vi "ExtractVINames.vi"(8 "error in (no error)":errorcluster, 11 "vi paths":string[](array[string])) -> (0 "error out":errorcluster, 3 "vi names":string[](array[string]))   [LabVIEW 2015, in "VeriStandTestUtilities.lvlib"]
uses:
  VeriStandTestUtilities.lvlib
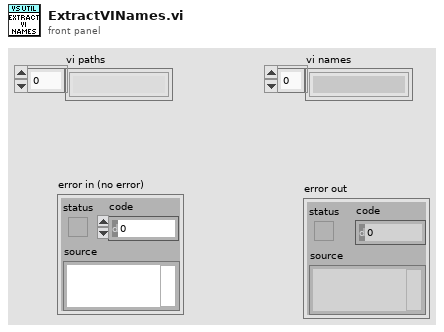
[diagram p1: front panel]
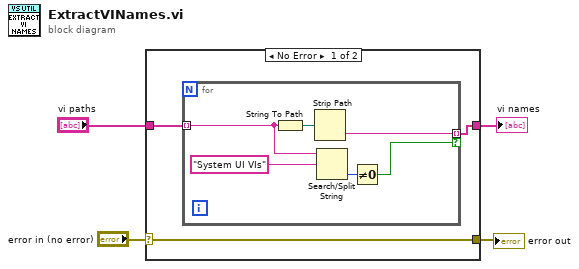
[diagram p0: block diagram]
diagram:
  n1 = case shown="No Error" "error in (no error)" {
    selector: "error in (no error)" -> [w5 w15]
    tunnel: [w5 w15] -> w4
    tunnel: "vi paths" -> [w7 w14]
    tunnel: [w6 w14] -> w1
    frame No Error {
      n2 = for {
        tunnel: w7 -> [w10] mode=indexing
        tunnel: [w9] -> w6 mode=indexing if=w8
        n3 = String To Path(string=w10) -> (path=w13:path)
        n4 = Strip Path(path=w13) -> (name=w9:string)  [unwired: 1 out]
        n5 = Search/Split String(string=w10, search string/char (-)="System UI VIs") -> (offset of match=w12:i32)  [unwired: 1 in, 2 out]
        n6 = Not Equal To 0?(x=w12) -> (x != 0?=w8:bool)
      }
    }
    frame Error {
    }
  }
  "error out" <- w4
  "vi names" <- w1
